vi "Send the Batman.vi"(8 "error in (no error)":errorcluster, 11 "Kasli Wrapper 2.0 in":refnum<class "Kasli Wrapper 2.0.lvclass">=refnum) -> (0 "error out":errorcluster, 3 "Kasli Wrapper 2.0 out":refnum<class "Kasli Wrapper 2.0.lvclass">)   [LabVIEW 2020, in "CIRCUS_uServices.lvlib" / "Kasli Wrapper 2.0.lvlib" / "Kasli Wrapper 2.0.lvclass"]
uses:
  Kasli Wrapper 2.0.lvclass
  TALOS/TALOS_PPL.lvlibp/Father of all uServices/Father of all uServices/Father of all uServices.lvclass
  TALOS/TALOS_PPL.lvlibp
  C:/Users/marco/Documents/GitHub_Lab/CIRCUS/TALOS/TALOS_PPL.lvlibp/Father of all uServices/Father of all uServices/Father of all uServices.lvclass
  C:/Users/marco/Documents/GitHub_Lab/CIRCUS/TALOS/TALOS_PPL.lvlibp/Ancestor/Ancestor/Ancestor.lvclass
  C:/Users/marco/Documents/GitHub_Lab/CIRCUS/TALOS/Actor Framework.lvlibp/1abvi3w/vi.lib/ActorFramework/Actor/Actor.lvclass
  C:/Users/marco/Documents/GitHub_Lab/CIRCUS/CIRCUS uServices et al/Kasli Wrapper 2.0/Kasli Wrapper 2.0.lvclass
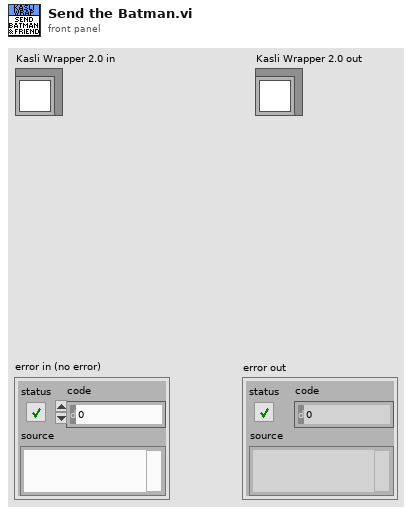
[diagram p1: front panel]
types:
  T1 = typedef "CIRCUS_uServices.lvlib/Run Utilities.lvlib/DAQ Control.ctl" = enum16{"On", "Off", "External"}
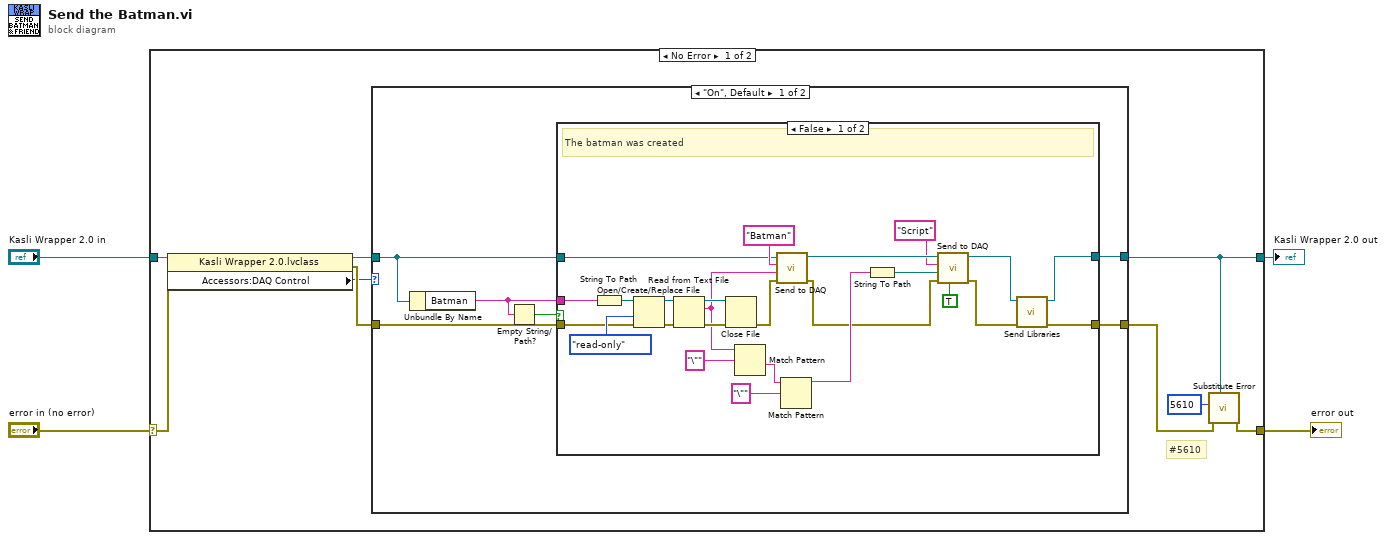
[diagram p0: block diagram]
diagram:
  n1 = case shown="No Error" "error in (no error)" {
    selector: "error in (no error)" -> [w11 w50]
    tunnel: [w8 w50] -> w4
    tunnel: "Kasli Wrapper 2.0 in" -> [w13 w49]
    tunnel: [w6 w49] -> w1
    frame No Error {
      # "#5610"
      n2 = property class="Kasli Wrapper 2.0.lvclass"(reference=w13, error in=w11) -> (reference out=w12:refnum<class "Kasli Wrapper 2.0.lvclass">, error out=w10:errorcluster, "Accessors:DAQ Control"=w5:T1)
      n3 = case shown="\"On\", Default" w5 {
        tunnel: w12 -> [w19 w47]
        tunnel: w10 -> [w18 w48]
        tunnel: [w17 w48] -> w9
        tunnel: [w16 w47] -> w6
        frame "On", Default {
          n4 = Unbundle By Name(w19) -> ("Batman"=w15:string)
          n5 = Empty String/Path?(string/path=w15) -> (empty?=w14:bool)
          n6 = case shown="False" w14 {
            tunnel: w15 -> [w44 _]
            tunnel: w19 -> [w41 w46]
            tunnel: w18 -> [w34 w45]
            tunnel: [w24 w45] -> w17
            tunnel: [w22 w46] -> w16
            frame False {
              # "The batman was created"
              n7 = String To Path(string=w44) -> (path=w36:path)
              n8 = Open/Create/Replace File(file path (use dialog)=w36, error in=w34, access (0:read/write)=enum16{"read/write", "read-only", "write-only"}."read-only") -> (refnum out=w39:refnum<file>, error out=w40:errorcluster)  [unwired: 3 in, 1 out]
              n9 = Read from Text File(file (use dialog)=w39, error in=w40) -> (refnum out=w38:refnum<file>, text=w30:string, error out=w37:errorcluster)  [unwired: 2 in, 1 out]
              n10 = Close File(refnum=w38, error in=w37) -> (error out=w27:errorcluster)  [unwired: 1 out]
              n11 = Match Pattern(string=w30, regular expression="\"") -> (after substring=w32:string)  [unwired: 1 in, 3 out]
              n12 = call "Send to DAQ.vi"("error in (no error)"=w27, "Data"=w30, "Data Name"="Batman", "Father of all uServices in"=w41) -> ("error out"=w26:errorcluster, "Father of all uServices out"=w42:refnum<class "Kasli Wrapper 2.0.lvclass">)  [unwired: 6 in]
              n13 = Match Pattern(string=w32, regular expression="\"") -> (before substring=w29:string)  [unwired: 1 in, 3 out]
              n14 = String To Path(string=w29) -> (path=w28:path)
              n15 = call "Send to DAQ.vi"("File?"=TRUE, "error in (no error)"=w26, "Data"=w28, "Data Name"="Script", "Father of all uServices in"=w42) -> ("error out"=w25:errorcluster, "Father of all uServices out"=w23:refnum<class "Kasli Wrapper 2.0.lvclass">)  [unwired: 5 in]
              n16 = call-dynamic "Send Libraries.vi"("error in (no error)"=w25, "Kasli Wrapper 2.0 in"=w23) -> ("error out"=w24:errorcluster, "Kasli Wrapper 2.0 out"=w22:refnum<class "Kasli Wrapper 2.0.lvclass">)  [unwired: 8 in]
            }
            frame True {
              # "Empty Batman = this Kasli didn't submit any script"
            }
          }
        }
        frame "Off" {
        }
      }
      n17 = call "Substitute Error.vi"("LabVIEW Object"=w6, "error in (no error)"=w9, "Error Code"=5610) -> ("error out"=w8:errorcluster)  [unwired: 8 in]
    }
    frame Error {
    }
  }
  "error out" <- w4
  "Kasli Wrapper 2.0 out" <- w1
